vi "Convert From JSON Comp Format.vi"(3 "output settings JSON":T1={"output rate"=51200.0, "range"=5.0, "terminal configuration"="", "output impedance"=0.0, "common mode offset"=0.0, "pure tone mode"=FALSE}, 8 "error in (no error)":errorcluster) -> (0 "error out":errorcluster, 11 "output settings":T2={"output rate"=51200.0, "range"=5.0, "terminal configuration"=enum."Pseudodifferential", "output impedance"=0.0, "common mode offset"=0.0, "pure tone mode"=FALSE})   [LabVIEW 2022 SP3, in "Analog Gen Settings.lvlib"]
uses:
  Analog Gen Settings.lvlib
  service/generation/controls/analog output settings.ctl
  service/generation/controls/terminal configuration.ctl
  analog output settings_json.ctl
  service/generation/controls/AudioGenTypeDefs.lvlib
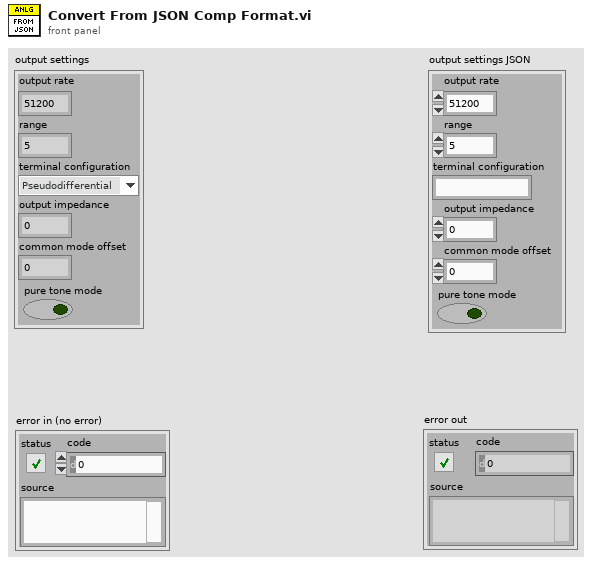
[diagram p1: front panel]
types:
  T1 = typedef "Analog Gen Settings.lvlib/analog output settings_json.ctl" = cluster{"output rate":dbl, "range":dbl, "terminal configuration":string, "output impedance":dbl, "common mode offset":dbl, "pure tone mode":bool}
  T2 = typedef "AudioGenTypeDefs.lvlib/analog output settings.ctl" = cluster{"output rate":dbl, "range":dbl, "terminal configuration":T3, "output impedance":dbl, "common mode offset":dbl, "pure tone mode":bool}
  T3 = typedef "AudioGenTypeDefs.lvlib/terminal configuration.ctl" = enum32{"Default", "RSE", "Differential", "Pseudodifferential"}
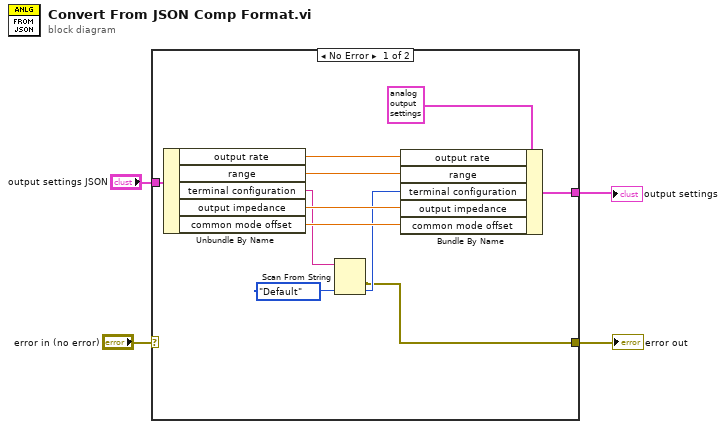
[diagram p0: block diagram]
diagram:
  n1 = case shown="No Error" "error in (no error)" {
    selector: "error in (no error)" -> [_ w16]
    tunnel: [w10 _] -> w4
    tunnel: "output settings JSON" -> [w9 _]
    tunnel: [w5 w16] -> w1
    frame No Error {
      n2 = Unbundle By Name(w9) -> ("output rate"=w15:dbl, "range"=w14:dbl, "terminal configuration"=w8:string, "output impedance"=w13:dbl, "common mode offset"=w12:dbl)
      n3 = Scan From String(input string=w8, default 1=terminal_configuration."Default" ("terminal configuration")) -> (error out=w5:errorcluster, output 1=w6:T3)  [unwired: 3 in, 2 out]
      n4 = Bundle By Name(cluster=T2 {"output rate"=51200.0, "range"=5.0, "terminal configuration"=enum."Pseudodifferential", "output impedance"=0.0, "common mode offset"=0.0, "pure tone mode"=FALSE} ("output settings"), "output rate"=w15, "range"=w14, "terminal configuration"=w6, "output impedance"=w13, "common mode offset"=w12) -> (w10:T2)
    }
    frame Error {
    }
  }
  "output settings" <- w4
  "error out" <- w1
